vi "PathPlanner_Path_MirrorPath.vi"(11 "in PathPlannerPath":T1={"Reversed"=FALSE, "RotationTargets"=[], "ConstraintZones"=[], "EventMarkers"=[], "GlobalConstraints"={"MaxVelocityMps;"=0.0, "MaxAccelerationMpsSq;"=0.0, "MaxAngularVelRadPsEc;"=0.0, "MaxAngularAccRadPSecSq"=0.0, "Exists"=FALSE, "Unlimited"=FALSE, "NominalVoltageVolts"=12.0}, "GoalEndState"={"VelocityMPS"=0.0, "Rotation"={"VALUE"=0.0, "COS"=1.0, "SIN"=0.0}}, "AllPoints"=[], "Name"="", "Waypoints"=[], "PointTowardsZones"=[], "IdealStartingState"={"VelocityMPS"=0.0, "Rotation"={"VALUE"=1.0, "COS"=0.0, "SIN"=0.0}, "NotNull"=FALSE}, "IsChoreoPath"=FALSE, "PreventFlipping"=FALSE} {"IdealStartingState"."Rotation"."SIN" format="%13.4f"; "IdealStartingState"."Rotation"."COS" format="%13.4f"; "IdealStartingState"."Rotation"."VALUE" format="%13.4f"; "PointTowardsZones"."TargetPosition"."Y" format="%14.3f"; "PointTowardsZones"."TargetPosition"."X" format="%14.3f"; "PointTowardsZones"."RotationOffset"."SIN" format="%13.4f"; "PointTowardsZones"."RotationOffset"."COS" format="%13.4f"; "PointTowardsZones"."RotationOffset"."VALUE" format="%13.4f"; "Waypoints"."nextControl"."Y" format="%14.3f"; "Waypoints"."nextControl"."X" format="%14.3f"; "Waypoints"."anchor"."Y" format="%14.3f"; "Waypoints"."anchor"."X" format="%14.3f"; "Waypoints"."prevControl"."Y" format="%14.3f"; "Waypoints"."prevControl"."X" format="%14.3f"; "AllPoints"."RotationTarget"."rotation"."SIN" format="%13.4f"; "AllPoints"."RotationTarget"."rotation"."COS" format="%13.4f"; "AllPoints"."RotationTarget"."rotation"."VALUE" format="%13.4f"; "AllPoints"."Position"."Y" format="%14.3f"; "AllPoints"."Position"."X" format="%14.3f"; "GoalEndState"."Rotation"."SIN" format="%13.4f"; "GoalEndState"."Rotation"."COS" format="%13.4f"; "GoalEndState"."Rotation"."VALUE" format="%13.4f"; "RotationTargets"."rotation"."SIN" format="%13.4f"; "RotationTargets"."rotation"."COS" format="%13.4f"; "RotationTargets"."rotation"."VALUE" format="%13.4f"}) -> (3 "out PathPlannerPath":T1={"Reversed"=FALSE, "RotationTargets"=[], "ConstraintZones"=[], "EventMarkers"=[], "GlobalConstraints"={"MaxVelocityMps;"=0.0, "MaxAccelerationMpsSq;"=0.0, "MaxAngularVelRadPsEc;"=0.0, "MaxAngularAccRadPSecSq"=0.0, "Exists"=FALSE, "Unlimited"=FALSE, "NominalVoltageVolts"=12.0}, "GoalEndState"={"VelocityMPS"=0.0, "Rotation"={"VALUE"=0.0, "COS"=1.0, "SIN"=0.0}}, "AllPoints"=[], "Name"="", "Waypoints"=[], "PointTowardsZones"=[], "IdealStartingState"={"VelocityMPS"=0.0, "Rotation"={"VALUE"=1.0, "COS"=0.0, "SIN"=0.0}, "NotNull"=FALSE}, "IsChoreoPath"=FALSE, "PreventFlipping"=FALSE} {"IdealStartingState"."Rotation"."SIN" format="%13.4f"; "IdealStartingState"."Rotation"."COS" format="%13.4f"; "IdealStartingState"."Rotation"."VALUE" format="%13.4f"; "PointTowardsZones"."TargetPosition"."Y" format="%14.3f"; "PointTowardsZones"."TargetPosition"."X" format="%14.3f"; "PointTowardsZones"."RotationOffset"."SIN" format="%13.4f"; "PointTowardsZones"."RotationOffset"."COS" format="%13.4f"; "PointTowardsZones"."RotationOffset"."VALUE" format="%13.4f"; "Waypoints"."nextControl"."Y" format="%14.3f"; "Waypoints"."nextControl"."X" format="%14.3f"; "Waypoints"."anchor"."Y" format="%14.3f"; "Waypoints"."anchor"."X" format="%14.3f"; "Waypoints"."prevControl"."Y" format="%14.3f"; "Waypoints"."prevControl"."X" format="%14.3f"; "AllPoints"."RotationTarget"."rotation"."SIN" format="%13.4f"; "AllPoints"."RotationTarget"."rotation"."COS" format="%13.4f"; "AllPoints"."RotationTarget"."rotation"."VALUE" format="%13.4f"; "AllPoints"."Position"."Y" format="%14.3f"; "AllPoints"."Position"."X" format="%14.3f"; "GoalEndState"."Rotation"."SIN" format="%13.4f"; "GoalEndState"."Rotation"."COS" format="%13.4f"; "GoalEndState"."Rotation"."VALUE" format="%13.4f"; "RotationTargets"."rotation"."SIN" format="%13.4f"; "RotationTargets"."rotation"."COS" format="%13.4f"; "RotationTargets"."rotation"."VALUE" format="%13.4f"})   [LabVIEW 2019, in "PathPlanner24.lvlib"]
doc: "Mirror a path to the other side of the current alliance. For example, if this path is on the right of the blue alliance side of the field, it will be mirrored to the left of the blue alliance side of the field.\n\n\nInputs: \n - Path - cluster - path definition data structure\n\nOutputs:\n - Path - cluster - mirrored path"
uses:
  PathPlanner24.lvlib
  <vilib>/Rock Robotics/WPI/ThirdParty/JAS_Junk/TrajLib/Trajectory_Library.lvlib
  <vilib>/Rock Robotics/WPI/ThirdParty/JAS_Junk/TrajLib/TypeDef/TRANSLATION2D.ctl
  <vilib>/Rock Robotics/WPI/ThirdParty/JAS_Junk/TrajLib/TypeDef/ROTATION2D.ctl
  TypeDef/PathPlannerPathConstraints.ctl
  TypeDef/PathPlannerRotationTarget.ctl
  TypeDef/PathPlannerConstraintsZone.ctl
  TypeDef/PathPlannerEventMarker.ctl
  TypeDef/PathPlannerGoalEndState.ctl
  TypeDef/PathPlannerPathPoint.ctl
  TypeDef/PathPlannerPath.ctl
  TypeDef/PathPlannerCommandUtil.ctl
  TypeDef/PathPlannerWaypoint.ctl
  TypeDef/PathPlannerPointTowardsZone.ctl
  TypeDef/PathPlannerIdealStartingState.ctl
  ENum/PathPlanner_CommandUtil_Type_ENUM.ctl
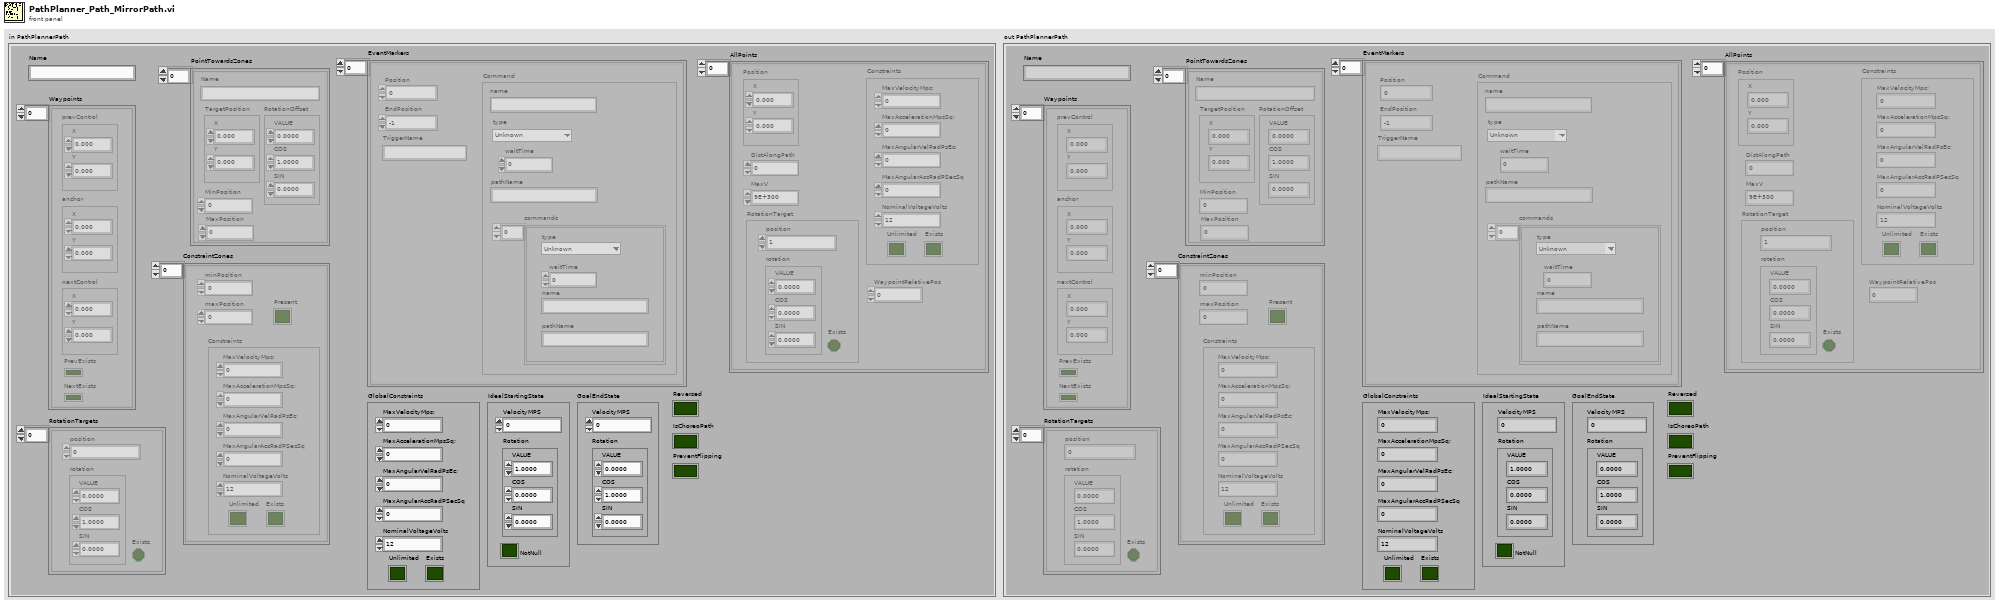
[diagram p1: front panel]
types:
  T1 = typedef "PathPlanner24.lvlib/PathPlannerPath.ctl" = cluster{"Reversed":bool, "RotationTargets":T2[], "ConstraintZones":T4[], "EventMarkers":T6[], "GlobalConstraints":T5, "GoalEndState":T9, "AllPoints":T10[], "Name":string, "Waypoints":T12[], "PointTowardsZones":T13[], "IdealStartingState":T14, "IsChoreoPath":bool, "PreventFlipping":bool}
  T2 = typedef "PathPlanner24.lvlib/PathPlannerRotationTarget.ctl" = cluster{"position":dbl, "rotation":T3, "Exists":bool}
  T3 = typedef "Trajectory_Library.lvlib/ROTATION2D.ctl" = cluster{"VALUE":dbl, "COS":dbl, "SIN":dbl}
  T4 = typedef "PathPlanner24.lvlib/PathPlannerConstraintsZone.ctl" = cluster{"minPosition":dbl, "maxPosition":dbl, "Constraints":T5, "Present":bool}
  T5 = typedef "PathPlanner24.lvlib/PathPlannerPathConstraints.ctl" = cluster{"MaxVelocityMps;":dbl, "MaxAccelerationMpsSq;":dbl, "MaxAngularVelRadPsEc;":dbl, "MaxAngularAccRadPSecSq":dbl, "Exists":bool, "Unlimited":bool, "NominalVoltageVolts":dbl}
  T6 = typedef "PathPlanner24.lvlib/PathPlannerEventMarker.ctl" = cluster{"Position":dbl, "Command":T7, "TriggerName":string, "EndPosition":dbl}
  T7 = typedef "PathPlanner24.lvlib/PathPlannerCommandUtil.ctl" = cluster{"waitTime":dbl, "name":string, "pathName":string, "commands":cluster{"type":T8, "waitTime":dbl, "name":string, "pathName":string}[], "type":T8}
  T8 = typedef "PathPlanner24.lvlib/PathPlanner_CommandUtil_Type_ENUM.ctl" = enum16{"Unknown", "Wait", "Named", "Path", "Sequential", "Parallel", "Race", "Deadline", "PointTowardsZoneEnter", "PointTowardsZoneExit", "TriggerEventStart", "TriggerEventStop", "TriggerEventOneshot"}
  T9 = typedef "PathPlanner24.lvlib/PathPlannerGoalEndState.ctl" = cluster{"VelocityMPS":dbl, "Rotation":T3}
  T10 = typedef "PathPlanner24.lvlib/PathPlannerPathPoint.ctl" = cluster{"Position":T11, "DistAlongPath":dbl, "MaxV":dbl, "Constraints":T5, "RotationTarget":T2, "WaypointRelativePos":dbl}
  T11 = typedef "Trajectory_Library.lvlib/TRANSLATION2D.ctl" = cluster{"X":dbl, "Y":dbl}
  T12 = typedef "PathPlanner24.lvlib/PathPlannerWaypoint.ctl" = cluster{"prevControl":T11, "anchor":T11, "nextControl":T11, "PrevExists":bool, "NextExists":bool}
  T13 = typedef "PathPlanner24.lvlib/PathPlannerPointTowardsZone.ctl" = cluster{"RotationOffset":T3, "Name":string, "TargetPosition":T11, "MinPosition":dbl, "MaxPosition":dbl}
  T14 = typedef "PathPlanner24.lvlib/PathPlannerIdealStartingState.ctl" = cluster{"VelocityMPS":dbl, "Rotation":T3, "NotNull":bool}
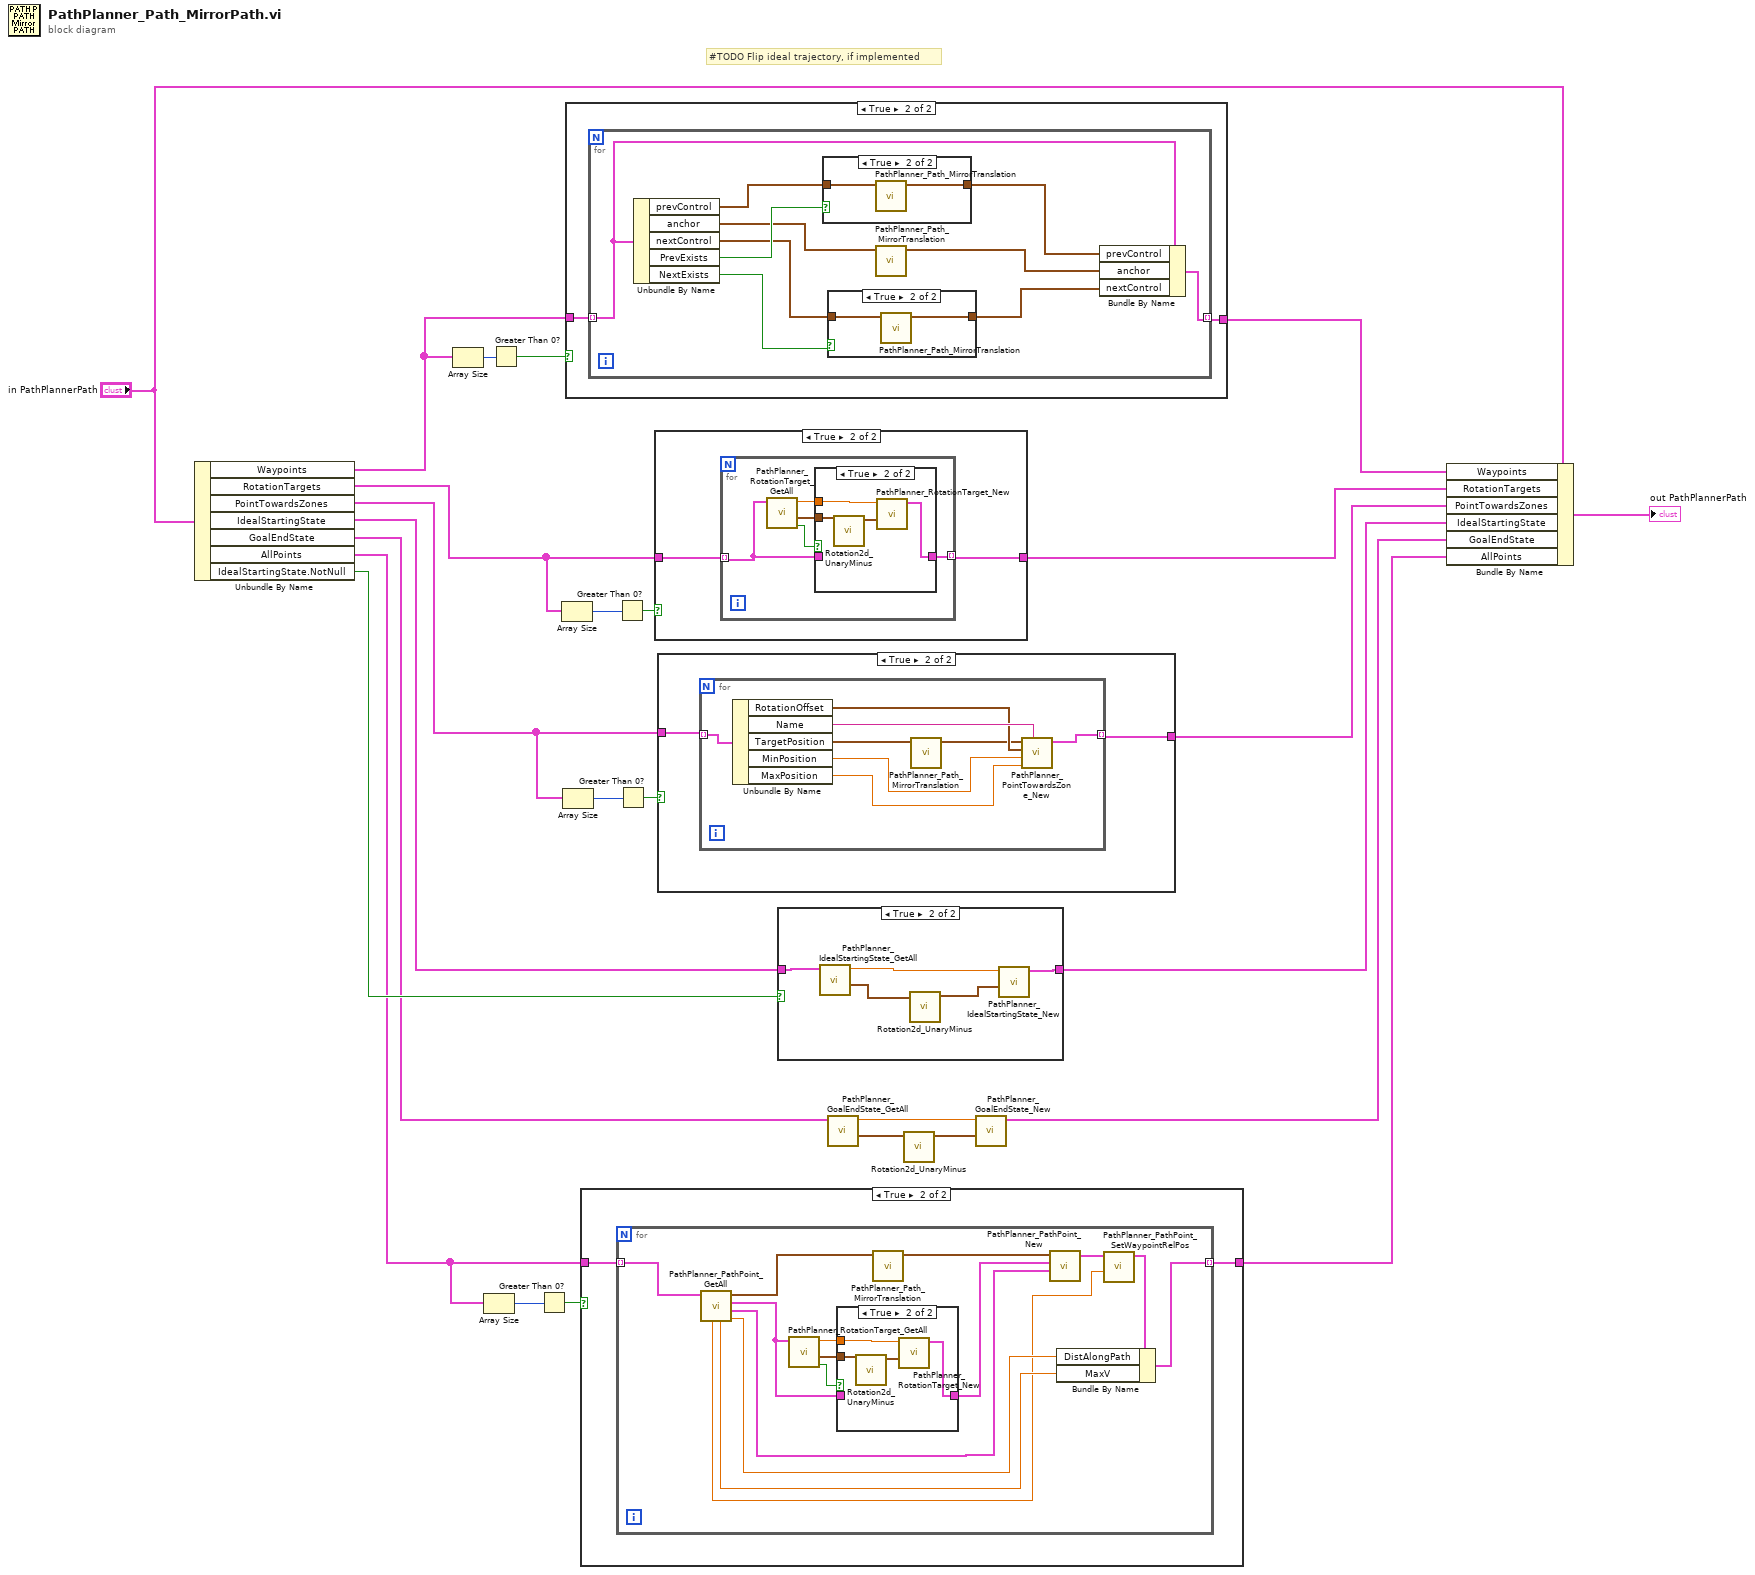
[diagram p0: block diagram]
diagram:
  # "#TODO Flip ideal trajectory, if implemented"
  n1 = Unbundle By Name("in PathPlannerPath") -> ("Waypoints"=w15:T12[], "RotationTargets"=w12:T2[], "PointTowardsZones"=w9:T13[], "IdealStartingState"=w21:T14, "GoalEndState"=w8:T9, "AllPoints"=w2:T10[], "IdealStartingState.NotNull"=w18:bool)
  n2 = Array Size(array=w15) -> (size(s)=w17:i32)
  n3 = Array Size(array=w2) -> (size(s)=w3:i32)
  n4 = Greater Than 0?(x=w17) -> (x > 0?=w16:bool)
  n5 = Greater Than 0?(x=w3) -> (x > 0?=w1:bool)
  n6 = Array Size(array=w12) -> (size(s)=w14:i32)
  n7 = Array Size(array=w9) -> (size(s)=w11:i32)
  n8 = case shown="True" w16 {
    tunnel: w15 -> [w27 w29]
    tunnel: [w27 w28] -> w24
    frame False {
    }
    frame True {
      n9 = for {
        tunnel: w29 -> [w39] mode=indexing
        tunnel: [w38] -> w28 mode=indexing
        n10 = Unbundle By Name(w39) -> ("prevControl"=w35:T11, "anchor"=w34:T11, "nextControl"=w33:T11, "PrevExists"=w37:bool, "NextExists"=w36:bool)
        n11 = case shown="True" w37 {
          tunnel: w35 -> [w43 w45]
          tunnel: [w43 w44] -> w30
          frame False {
          }
          frame True {
            n12 = call "PathPlanner_Path_MirrorTranslation.vi"("inTranslation"=w45) -> ("MirrorTranslation"=w44:T11)  [unwired: 10 in]
          }
        }
        n13 = case shown="True" w36 {
          tunnel: w33 -> [w40 w42]
          tunnel: [w40 w41] -> w32
          frame False {
          }
          frame True {
            n14 = call "PathPlanner_Path_MirrorTranslation.vi"("inTranslation"=w42) -> ("MirrorTranslation"=w41:T11)  [unwired: 10 in]
          }
        }
        n15 = call "PathPlanner_Path_MirrorTranslation.vi"("inTranslation"=w34) -> ("MirrorTranslation"=w31:T11)  [unwired: 10 in]
        n16 = Bundle By Name(cluster=w39, "prevControl"=w30, "anchor"=w31, "nextControl"=w32) -> (w38:T12)
      }
    }
  }
  n17 = case shown="True" w1 {
    tunnel: [w46 w48] -> w19
    tunnel: w2 -> [w46 w47]
    frame False {
    }
    frame True {
      n18 = for {
        tunnel: w47 -> [w63] mode=indexing
        tunnel: [w58] -> w48 mode=indexing
        n19 = call "PathPlanner_PathPoint_GetAll.vi"("PathPlannerPoint"=w63) -> ("DistAlongPath"=w51:dbl, "Constraints"=w52:T5, "RotationTarget"=w54:T2, "Position"=w61:T11, "MaxV"=w50:dbl, "WaypointRelativePos"=w49:dbl)  [unwired: 5 in]
        n20 = call "PathPlanner_RotationTarget_GetAll.vi"("RotationTarget"=w54) -> ("Exists"=w56:bool, "rotation"=w55:T3, "position"=w57:dbl)  [unwired: 8 in]
        n21 = case shown="True" w56 {
          tunnel: w57 -> [_ w68]
          tunnel: w55 -> [_ w66]
          tunnel: [w64 w65] -> w53
          tunnel: w54 -> [w64 _]
          frame False {
          }
          frame True {
            n22 = call <vilib>:"Rotation2d_UnaryMinus.vi"("in ROTATION"=w66) -> ("out ROTATION"=w67:T3)  [unwired: 10 in]
            n23 = call "PathPlanner_RotationTarget_New.vi"("rotation"=w67, "position"=w68) -> ("RotationTarget"=w65:T2)  [unwired: 9 in]
          }
        }
        n24 = call "PathPlanner_Path_MirrorTranslation.vi"("inTranslation"=w61) -> ("MirrorTranslation"=w60:T11)  [unwired: 10 in]
        n25 = call "PathPlanner_PathPoint_New.vi"("Constraints"=w52, "RotationTarget"=w53, "Position"=w60) -> ("PathPlannerPoint"=w62:T10)  [unwired: 8 in]
        n26 = call "PathPlanner_PathPoint_SetWaypointRelPos.vi"("WaypointRelativePos"=w49, "PathPlannerPoint"=w62) -> ("outPathPlannerPoint"=w59:T10)  [unwired: 9 in]
        n27 = Bundle By Name(cluster=w59, "DistAlongPath"=w51, "MaxV"=w50) -> (w58:T10)
      }
    }
  }
  n28 = Greater Than 0?(x=w14) -> (x > 0?=w13:bool)
  n29 = Greater Than 0?(x=w11) -> (x > 0?=w10:bool)
  n30 = case shown="True" w13 {
    tunnel: w12 -> [w69 w71]
    tunnel: [w69 w70] -> w23
    frame False {
    }
    frame True {
      n31 = for {
        tunnel: w71 -> [w72] mode=indexing
        tunnel: [w73] -> w70 mode=indexing
        n32 = call "PathPlanner_RotationTarget_GetAll.vi"("RotationTarget"=w72) -> ("Exists"=w75:bool, "rotation"=w74:T3, "position"=w76:dbl)  [unwired: 8 in]
        n33 = case shown="True" w75 {
          tunnel: w76 -> [_ w81]
          tunnel: w74 -> [_ w79]
          tunnel: [w77 w78] -> w73
          tunnel: w72 -> [w77 _]
          frame False {
          }
          frame True {
            n34 = call <vilib>:"Rotation2d_UnaryMinus.vi"("in ROTATION"=w79) -> ("out ROTATION"=w80:T3)  [unwired: 10 in]
            n35 = call "PathPlanner_RotationTarget_New.vi"("rotation"=w80, "position"=w81) -> ("RotationTarget"=w78:T2)  [unwired: 9 in]
          }
        }
      }
    }
  }
  n36 = case shown="True" w10 {
    tunnel: w9 -> [w82 w84]
    tunnel: [w82 w83] -> w22
    frame False {
    }
    frame True {
      n37 = for {
        tunnel: w84 -> [w92] mode=indexing
        tunnel: [w85] -> w83 mode=indexing
        n38 = Unbundle By Name(w92) -> ("RotationOffset"=w90:T3, "Name"=w91:string, "TargetPosition"=w89:T11, "MinPosition"=w87:dbl, "MaxPosition"=w86:dbl)
        n39 = call "PathPlanner_Path_MirrorTranslation.vi"("inTranslation"=w89) -> ("MirrorTranslation"=w88:T11)  [unwired: 10 in]
        n40 = call "PathPlanner_PointTowardsZone_New.vi"("Name"=w91, "MaxPosition"=w86, "MinPosition"=w87, "RotationOffset"=w90, "TargetPosition"=w88) -> ("PointTowardsZone"=w85:T13)  [unwired: 6 in]
      }
    }
  }
  n41 = case shown="True" w18 {
    tunnel: w21 -> [w93 w97]
    tunnel: [w93 w98] -> w20
    frame False {
    }
    frame True {
      n42 = call "PathPlanner_IdealStartingState_GetAll.vi"("IdealStartingState"=w97) -> ("Rotation"=w95:T3, "VelocityMPS"=w96:dbl)  [unwired: 8 in, 1 out]
      n43 = call <vilib>:"Rotation2d_UnaryMinus.vi"("in ROTATION"=w95) -> ("out ROTATION"=w94:T3)  [unwired: 10 in]
      n44 = call "PathPlanner_IdealStartingState_New.vi"("Rotation"=w94, "VelocityMPS"=w96) -> ("IdealStartingState"=w98:T14)  [unwired: 9 in]
    }
  }
  n45 = call "PathPlanner_GoalEndState_GetAll.vi"("GoalEndState"=w8) -> ("Rotation"=w5:T3, "VelocityMPS"=w6:dbl)  [unwired: 9 in]
  n46 = call <vilib>:"Rotation2d_UnaryMinus.vi"("in ROTATION"=w5) -> ("out ROTATION"=w4:T3)  [unwired: 10 in]
  n47 = call "PathPlanner_GoalEndState_New.vi"("Rotation"=w4, "VelocityMPS"=w6) -> ("GoalEndState"=w7:T9)  [unwired: 9 in]
  n48 = Bundle By Name(cluster="in PathPlannerPath", "Waypoints"=w24, "RotationTargets"=w23, "PointTowardsZones"=w22, "IdealStartingState"=w20, "GoalEndState"=w7, "AllPoints"=w19) -> (→"out PathPlannerPath":T1)
